vi "AttrMap-Preview.vi"(8 "error in (no error)":errorcluster, 11 "AttrMap in":T1) -> (0 "error out":errorcluster, 2 "table":string[][](array[string]), 3 "AttrMap out":T1)   [LabVIEW 2019]
uses:
  Typedef/Def-AttrMap.ctl
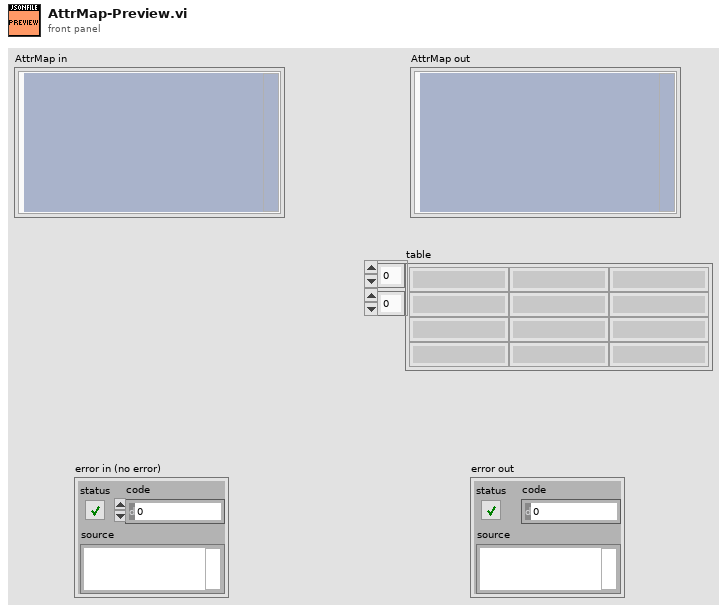
[diagram p1: front panel]
types:
  T1 = typedef "Def-AttrMap.ctl" = cluster{"Map":variant}
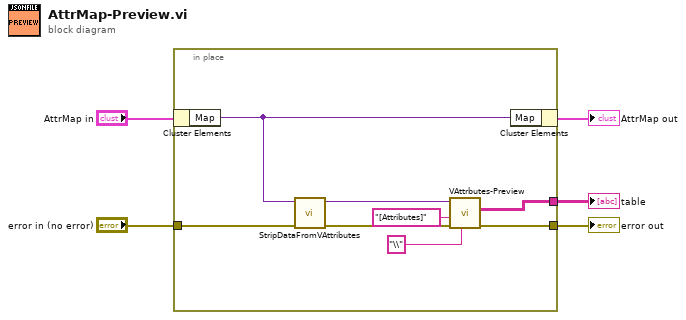
[diagram p0: block diagram]
diagram:
  n1 = in-place "In Place Element Structure" {
    in-place-border: [w8] -> w5
    in-place-border: "error in (no error)" -> [w12]
    in-place-border: [w7] -> w1
    n2 = in-place-cluster #1("AttrMap in") -> ("Map"=w13:variant)
    n3 = call "StripDataFromVAttributes.vi"("error in (no error)"=w12, "Map"=w13) -> ("error out"=w9:errorcluster, "duplicate variant"=w10:variant)  [unwired: 8 in]
    n4 = call "VAttrbutes-Preview.vi"("delimiter (/)"="\\", "error in"=w9, "ParentStr"="[Attributes]", "VAttributes"=w10) -> ("error out"=w8:errorcluster, "Array"=w7:string[][])  [unwired: 5 in, 1 out]
    n5 = in-place-cluster #1("Map"=w13) -> (→"AttrMap out":T1)
  }
  "error out" <- w5
  "table" <- w1
